vi "setUp.vi"(8 "error in (no error)":errorcluster, 11 "reference in":refnum<class "Test Network Stream Listener Connect.lvclass">) -> (0 "error out":errorcluster, 3 "reference out":refnum<class "Test Network Stream Listener Connect.lvclass">)   [LabVIEW 2020, in "Test Network Stream Listener Connect.lvclass"]
doc: "setUp runs prior to the test method during test execution. Use this method to initialize any object data required by your tests."
uses:
  Test Network Stream Listener Connect.lvclass
  <vilib>/addons/_JKI Toolkits/VI Tester/TestCase.llb/TestCase.lvclass
  Source/Protocols/Network Stream Strategy/Network Stream/Network Stream.lvclass
  Source/Protocols/Network Stream Strategy/Netowrk Stream Listener/Network Stream Listener.lvclass
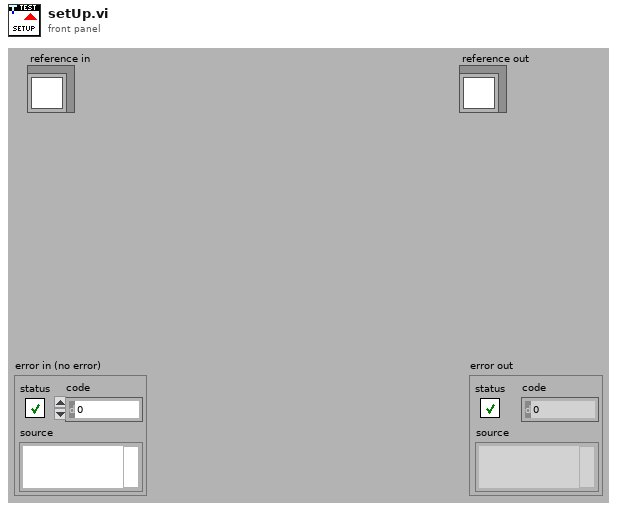
[diagram p1: front panel]
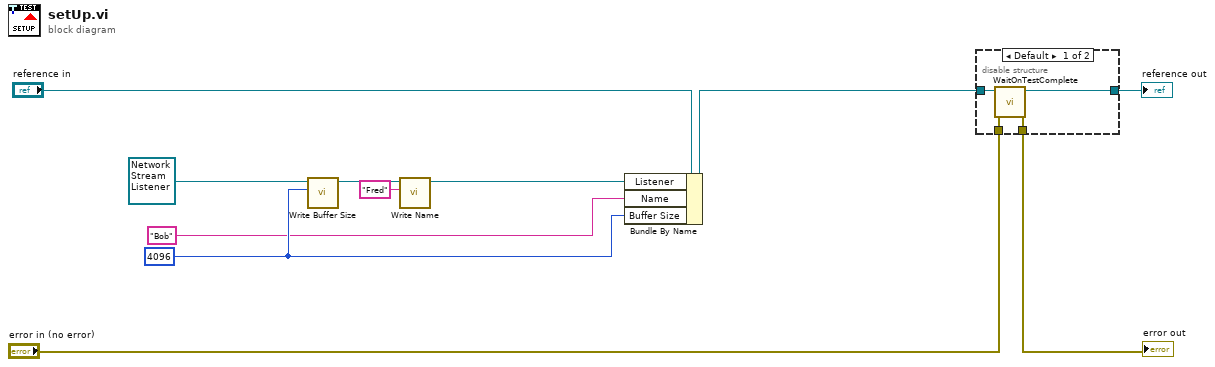
[diagram p0: block diagram]
diagram:
  w6 = 4096 ("Buffer Size")
  n1 = call "Write Buffer Size.vi"("Buffer Size"=w6, "Network Stream in"=refnum<class "Network Stream Listener.lvclass"> refnum ("Network Stream Listener.lvclass")) -> ("Network Stream out"=w5:refnum<class "Network Stream Listener.lvclass">)  [unwired: 9 in]
  n2 = call "Write Name.vi"("Name"="Fred", "Network Stream in"=w5) -> ("Network Stream out"=w4:refnum<class "Network Stream Listener.lvclass">)  [unwired: 9 in]
  n3 = Bundle By Name(cluster="reference in", "Listener"=w4, "Name"="Bob" ("Remote Name"), "Buffer Size"=w6) -> (w7:refnum<class "Test Network Stream Listener Connect.lvclass">)
  n4 = disable-structure shown="Default" {
    disable-tunnel: "error in (no error)" -> [w15 w16]
    disable-tunnel: [w14 w16] -> w10
    disable-tunnel: [w13 w17] -> w8
    disable-tunnel: w7 -> [w12 w17]
    frame condition #0 (active) {
      n5 = call <vilib>:"WaitOnTestComplete.vi"("error in (no error)"=w15, "TestCase in"=w12) -> ("error out"=w14:errorcluster, "TestCase out"=w13:refnum<class "Test Network Stream Listener Connect.lvclass">)  [unwired: 8 in]
    }
    frame condition #1 {
    }
  }
  "error out" <- w10
  "reference out" <- w8
